vi "Write Do.vi"(0 "FPGA API in":refnum<class "FPGA API Concrete.lvclass">, 5 "#DO":T1 items=["DO 0 [KP1] [M12]", "DO 1 [ON KP2] [M21]", "DO 2 [ON KP3] [M24]", "DO 3 [WATER Y18.1 [DO3]]", "DO 4 [WATER Y18.2 [DO4]]", "DO 5 [KP6 Y29.1 33.7]", "DO 6 [KP7 Y29.2 33.8]", "DO 7 [KP8 Y29.3 33.9]", "DO 8 [KP9 Y29.4  33.12]", "DO 9 [KP10 Y29.5 33.1]", "DO 10 [KP11 Y29.6 33.2]", "DO 11 [KP12 Y29.7  33.13]", "DO 12 [KP13 Y29.8  33.11]", "DO 13 [KP14 Y29.9 33.10]", "DO 14 [KP15 Y29.10  33.6]", "DO 15 [KP16 Y29.11  33.5]", "DO 16 [KP17 Y29.12  33.4]", "DO 17 [KP18 Y29.13 33.3]", "DO 18 [AIR KP19]", "DO 19 [STEP DRIVE EN KP20]", "DO 20 [KP21 Y44.1 OPEN]", "DO 21 [ KP22 Y44.1 CLOSE]", "DO 22 [ KP23 Y44.2 OPEN]", "DO 23", "DO 24 [STEP DRIVE 1]", "DO 25 [STEP DRIVE 2]"], 7 "value":bool, 9 "Time uSec":u32, 11 "error in (no error)":errorcluster) -> (4 "FPGA API out":refnum<class "FPGA API Concrete.lvclass">, 15 "error out":errorcluster)   [LabVIEW 2019, in "FPGA API Concrete.lvclass"]
uses:
  FPGA API Concrete.lvclass
  C:/Users/ANENKOV_V1/Desktop/src/FPGA_API_class/FPGA API.lvclass
  FPGA/TypeDef/DO index.ctl
  FPGA API Concrete.lvclass/FPGA API Concrete.ctl
  FPGA_API_class/FPGA API.lvclass/FPGA API.ctl
  <vilib>/Utility/error.llb/Error Cluster From Error Code.vi
  <vilib>/rvi/errors/niLvFpgaAdjustHostInterfaceError.vi
  <vilib>/rvi/interface/nirviMethod/nirviMethod.xnode
  FPGA Ref.ctl
  FPGA_API_class/FPGA API.lvclass
  <vilib>/FPGAPlugInAG/Dynamic/niLvFpga_WriteFifo_Dynamic.vi
  <vilib>/rvi/errors/niLvFpgaMergeErrorWithErrorCode.vi
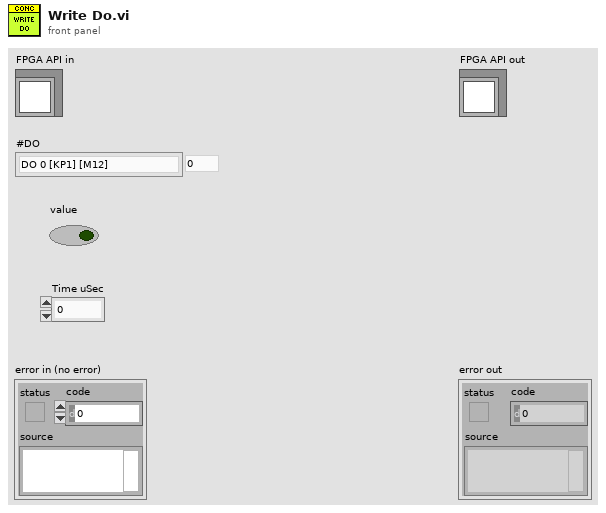
[diagram p1: front panel]
types:
  T1 = typedef "DO index.ctl" = u8
  T2 = typedef "FPGA API Concrete.lvclass/FPGA Ref.ctl" = refnum<k20>
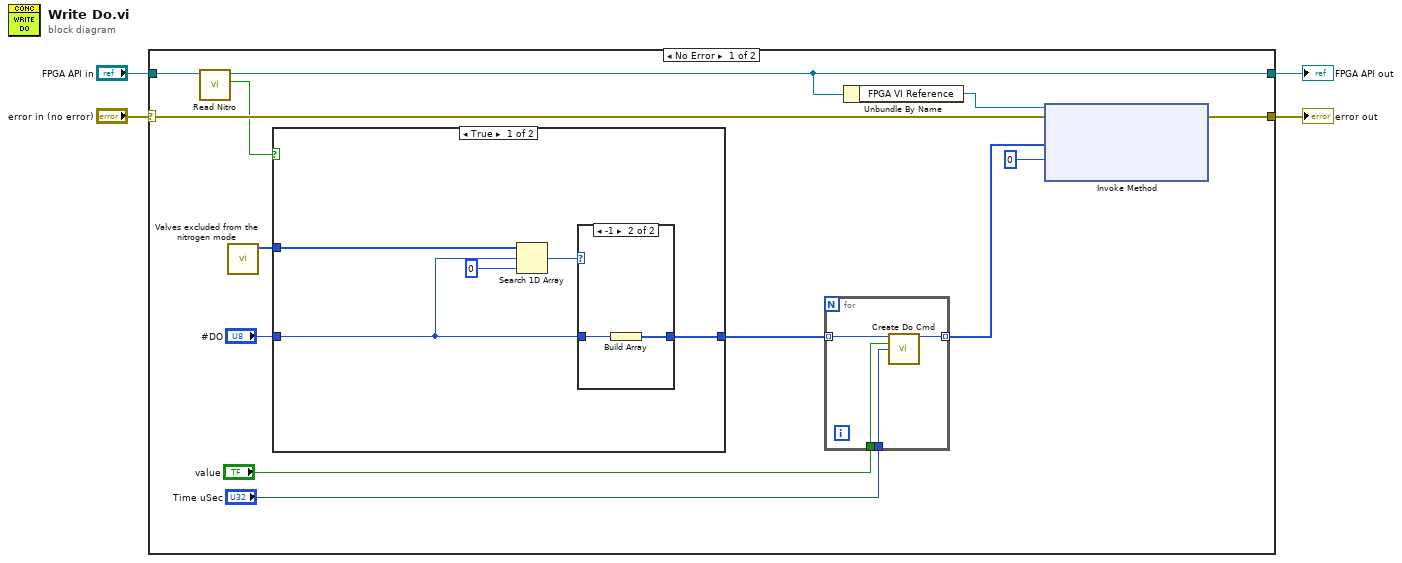
[diagram p0: block diagram]
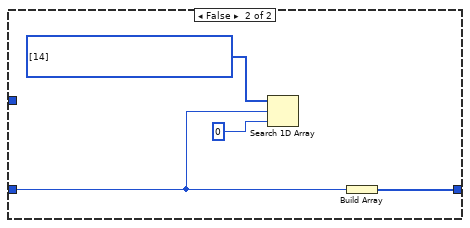
[diagram p3: hidden frame]
diagram:
  n1 = case shown="No Error" "error in (no error)" {
    selector: "error in (no error)" -> [w15 w34]
    tunnel: [w14 w34] -> w3
    tunnel: [w12 w33] -> w1
    tunnel: "FPGA API in" -> [w13 w33]
    frame No Error {
      n2 = call "Read Nitro.vi"("FPGA API in"=w13) -> ("Nitro"=w11:bool, "FPGA API out"=w12:refnum<class "FPGA API Concrete.lvclass">)  [unwired: 9 in]
      n3 = call "Valves excluded from the nitrogen mode.vi"() -> ("#DO"=w9:T1[])  [unwired: 11 in]
      n4 = case shown="True" w11 {
        tunnel: [w23 w30] -> w8
        tunnel: "#DO" -> [w24 w31]
        tunnel: w9 -> [w22 _]
        frame True {
          n5 = Search 1D Array(1D array=w22, element=w24, start index (0)=0) -> (index of element=w25:i32)
          n6 = case shown="-1" w25 {
            tunnel: w24 -> [_ w28]
            tunnel: [_ w27] -> w23
            frame Default {
            }
            frame -1 {
              n7 = Build Array(w28) -> (w27:T1[])
            }
          }
        }
        frame False {
          w29 = T1[] [14] items=["DO 0 [KP1] [M12]", "DO 1 [ON KP2] [M21]", "DO 2 [ON KP3] [M24]", "DO 3 [WATER Y18.1 [DO3]]", "DO 4 [WATER Y18.2 [DO4]]", "DO 5 [KP6 Y29.1 33.7]", "DO 6 [KP7 Y29.2 33.8]", "DO 7 [KP8 Y29.3 33.9]", "DO 8 [KP9 Y29.4  33.12]", "DO 9 [KP10 Y29.5 33.1]", "DO 10 [KP11 Y29.6 33.2]", "DO 11 [KP12 Y29.7  33.13]", "DO 12 [KP13 Y29.8  33.11]", "DO 13 [KP14 Y29.9 33.10]", "DO 14 [KP15 Y29.10  33.6]", "DO 15 [KP16 Y29.11  33.5]", "DO 16 [KP17 Y29.12  33.4]", "DO 17 [KP18 Y29.13 33.3]", "DO 18 [AIR KP19]", "DO 19 [STEP DRIVE EN KP20]", "DO 20 [KP21 Y44.1 OPEN]", "DO 21 [ KP22 Y44.1 CLOSE]", "DO 22 [ KP23 Y44.2 OPEN]", "DO 23", "DO 24 [STEP DRIVE 1]", "DO 25 [STEP DRIVE 2]"] ("1D array")
          n8 = Search 1D Array(1D array=w29, element=w31, start index (0)=0) -> ()  [unwired: 1 out]
          n9 = Build Array(w31) -> (w30:T1[])
        }
      }
      n10 = for {
        tunnel: w8 -> [w21] mode=indexing
        tunnel: [w20] -> w7 mode=indexing
        tunnel: "Time uSec" -> [w19]
        tunnel: "value" -> [w18]
        n11 = call "Create Do Cmd.vi"("#DO"=w21, "value"=w18, "Time uSec"=w19) -> ("Numeric"=w20:u64)  [unwired: 12 in]
      }
      n12 = Unbundle By Name(w12) -> ("FPGA VI Reference"=w16:T2)
      n13 = xnode "Invoke Method"("FPGA VI Reference In"=w16, "error in"=w15, "Data"=w7, "Timeout (ms)"=0) -> ("error out"=w14:errorcluster)  [unwired: 2 out]
    }
    frame Error {
    }
  }
  "error out" <- w3
  "FPGA API out" <- w1
